vi "PH_Powermeter_BaseClass.PC Write PSDB.vi"(0 "i ref in":refnum<vi>, 5 "error IO":errorcluster) -> (14 "i ref out":refnum<vi>, 17 "PSDB Numeric Data Array":T2[](array[typedef]), 18 "PSDB String Data Array":T1[](array[typedef]), 19 "error out":errorcluster)   [LabVIEW 2014, in "PH_Powermeter_BaseClass.lvlib"]
doc: "This is the proc case which writes data to the PHELIX shot data base."
uses:
  PH_Powermeter_BaseClass.lvlib
  PH_PSDBWriter/PH_PSDBWriter.Numeric dataset.ctl
  PH_PSDBWriter/PH_PSDBWriter.String dataset.ctl
  PH_PSDBWriter/PH_PSDBWriter.lvlib
  PH_StatusHandler/PH_StatusHandler.lvlib
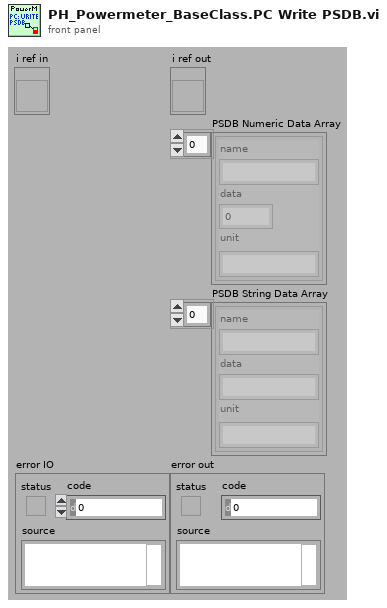
[diagram p1: front panel]
types:
  T1 = typedef "PH_PSDBWriter.lvlib/PH_PSDBWriter.String dataset.ctl" = cluster{"name":string, "data":string, "unit":string}
  T2 = typedef "PH_PSDBWriter.lvlib/PH_PSDBWriter.Numeric dataset.ctl" = cluster{"name":string, "data":dbl, "unit":string}
  T3 = typedef "PH_StatusHandler.lvlib/PH_StatusHandler.Status.ctl" = i16
  T4 = typedef "PH_Powermeter_BaseClass.lvlib/PH_Powermeter_BaseClass.i attribute.ctl" = cluster{"GUI References":T5, "Connection":T6, "Head Attributes":T8, "VISA resource":refnum<visa-resource-name>, "Energy":T9, "Service ID Energy":i32, "Wanted Settings":T10, "Current Settings":T10}
  T5 = typedef "PH_Powermeter_BaseClass.lvlib/PH_Powermeter_BaseClass.GUI Refs.ctl" = cluster{"Head Attributes":refnum<vi>, "Energy":refnum<vi>, "Connection":refnum<vi>, "VISA Resource":refnum<vi>, "Energy evolution":refnum<vi>, "Scaling Factor":refnum<vi>, "Range":refnum<vi>, "Wavelength":refnum<vi>, "Trigger Level":refnum<vi>, "Wanted Settings":refnum<vi>, "Current Settings":refnum<vi>}
  T6 = typedef "PH_Powermeter_BaseClass.lvlib/PH_Powermeter_BaseClass.Connection.ctl" = cluster{"failed checks":i8, "Timeout":bool, "Data read":string, "Failure":bool, "Error":bool, "State":T7}
  T7 = typedef "PH_Powermeter_BaseClass.lvlib/PH_Powermeter_BaseClass.State.ctl" = enum32{"off", "operating", "opened", "checked", "connected", "Sets to change", "running"}
  T8 = typedef "PH_Powermeter_BaseClass.lvlib/PH_Powermeter_BaseClass.Head Attributes.ctl" = cluster{"Instrument Type":string, "Head Version":string, "Head Name":string, "Serial Number":string, "Firmware":string, "Sensor Type":string, "MinimumRange":u32, "Maximum Range":u32, "Min Wavelength":i32, "Max Wavelength":i32}
  T9 = typedef "PH_Powermeter_BaseClass.lvlib/PH_Powermeter_BaseClass.Energy.ctl" = cluster{"current Value":dbl, "unscaled":dbl, "Scaling Factor":dbl}
  T10 = typedef "PH_Powermeter_BaseClass.lvlib/PH_gentec_BaseClass.Head Settings.ctl" = cluster{"Trigger Level":dbl, "Wavelength":u32, "Range":u32}
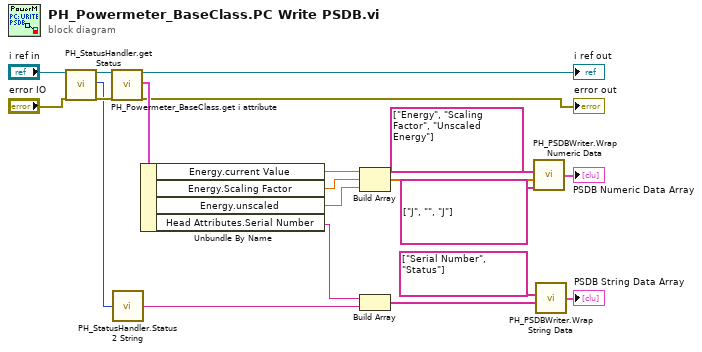
[diagram p0: block diagram]
diagram:
  n1 = call "PH_StatusHandler.get Status.vi"("VI in"="i ref in", "error in"="error IO") -> ("VI out"=w5:refnum<vi>, "Status"=w3:T3, "error out"=w4:errorcluster)  [unwired: 15 in]
  n2 = call "PH_Powermeter_BaseClass.get i attribute.vi"("i ref in"=w5, "error in (no error)"=w4) -> ("i ref out"=→"i ref out":refnum<vi>, "i attribute"=w20:T4, "error out"=→"error out":errorcluster)  [unwired: 15 in]
  n3 = call "PH_StatusHandler.Status 2 String.vi"("Status"=w3) -> ("Status as string"=w2:string)
  n4 = Unbundle By Name(w20) -> ("Energy.current Value"=w12:dbl, "Energy.Scaling Factor"=w19:dbl, "Energy.unscaled"=w1:dbl, "Head Attributes.Serial Number"=w13:string)
  n5 = Build Array(w12, w19, w1) -> (w15:dbl[])
  n6 = Build Array(w13, w2) -> (w17:string[])
  n7 = call "PH_PSDBWriter.Wrap Numeric Data.vi"("Unit Array"=string[] ["J", "", "J"], "Data Array"=w15, "Name Array"=string[] ["Energy", "Scaling Factor", "Unscaled Energy"]) -> ("PSDB Numeric Data Array"=→"PSDB Numeric Data Array":T2[])  [unwired: 1 in]
  n8 = call "PH_PSDBWriter.Wrap String Data.vi"("Data Array"=w17, "Name Array"=string[] ["Serial Number", "Status"]) -> ("PSDB String Data Array"=→"PSDB String Data Array":T1[])  [unwired: 2 in]
